vi "Simulation-4 (Case Control)_B220061.vi"() -> ()   [LabVIEW 2021]
panel:
  out "x-y":dbl
  in  "y":dbl
  in  "x":dbl
  out "x+y":dbl
  in  "Boolean":bool
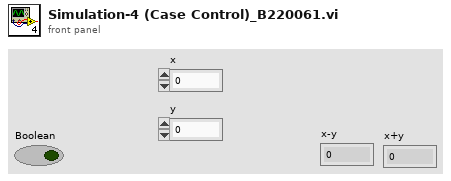
[diagram p1: front panel]
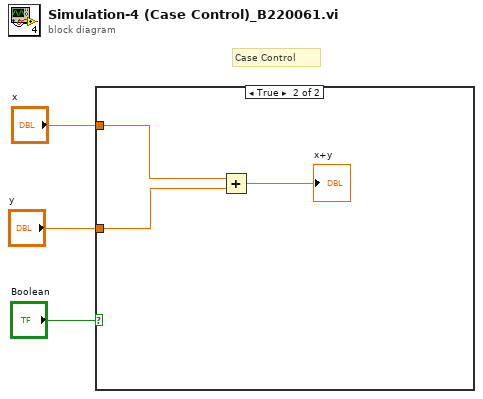
[diagram p0: block diagram]
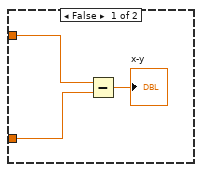
[diagram p2: hidden frame]
diagram:
  # "Case Control"
  n1 = case shown="True" "Boolean" {
    tunnel: "x" -> [w5 w8]
    tunnel: "y" -> [w4 w7]
    frame False {
      n2 = Subtract(x=w5, y=w4) -> (x-y=→"x-y":dbl)
    }
    frame True {
      n3 = Add(x=w8, y=w7) -> (x+y=→"x+y":dbl)
    }
  }
